vi "Write NumberOfRobots.vi"(8 "error in (no error)":errorcluster, 10 "NumberOfRobots":dbl, 11 "FreeBallPlayVSS in":refnum<class "FreeBallPlayVSS.lvclass">) -> (0 "error out":errorcluster, 3 "FreeBallPlayVSS out":refnum<class "FreeBallPlayVSS.lvclass">)   [LabVIEW 2023, in "FreeBallPlayVSS.lvclass"]
uses:
  FreeBallPlayVSS.lvclass
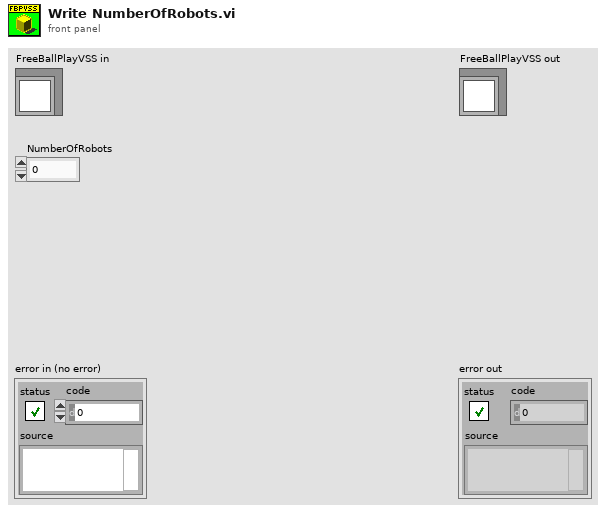
[diagram p1: front panel]
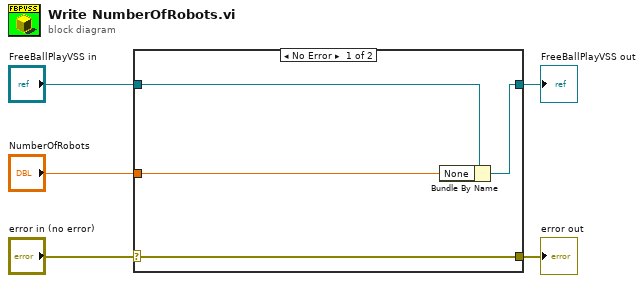
[diagram p0: block diagram]
diagram:
  n1 = case shown="No Error" "error in (no error)" {
    selector: "error in (no error)" -> [w9 w10]
    tunnel: [w9 w10] -> w4
    tunnel: [w7 w11] -> w2
    tunnel: "FreeBallPlayVSS in" -> [w8 w11]
    tunnel: "NumberOfRobots" -> [w6 _]
    frame No Error {
      n2 = Bundle By Name(cluster=w8, "None"=w6) -> (w7:refnum<class "FreeBallPlayVSS.lvclass">)
    }
    frame Error {
    }
  }
  "error out" <- w4
  "FreeBallPlayVSS out" <- w2
